vi "Read B.vi"(8 "Error In":errorcluster, 11 "NumericOperation in":refnum<class "NumericOperation.lvclass">) -> (0 "Error Out":errorcluster, 2 "B":dbl, 3 "NumericOperation out":refnum<class "NumericOperation.lvclass">)   [LabVIEW 2021, in "Calculator.lvlib" / "NumericOperation.lvclass"]
uses:
  NumericOperation.lvclass
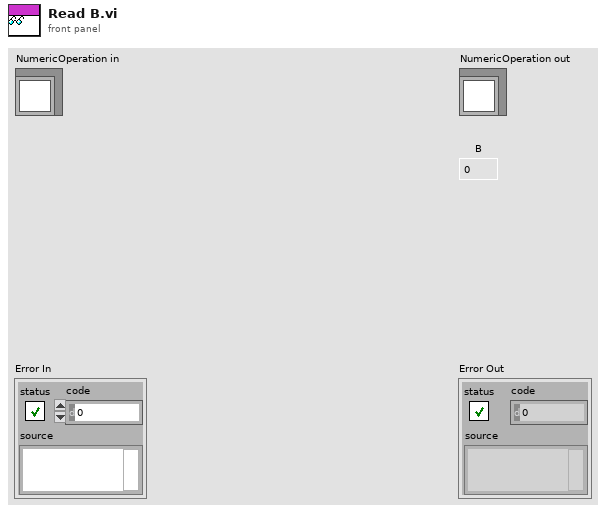
[diagram p1: front panel]
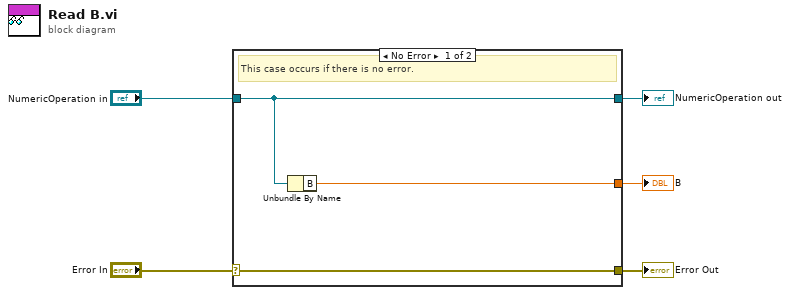
[diagram p0: block diagram]
diagram:
  n1 = case shown="No Error" "Error In" {
    selector: "Error In" -> [w8 w9]
    tunnel: [w8 w9] -> w4
    tunnel: [w7 w10] -> w2
    tunnel: "NumericOperation in" -> [w7 w10]
    tunnel: [w6 _] -> w1
    frame No Error {
      # "This case occurs if there is no error."
      n2 = Unbundle By Name(w7) -> ("B"=w6:dbl)
    }
    frame Error {
      # "This case occurs if there is any error"
    }
  }
  "Error Out" <- w4
  "NumericOperation out" <- w2
  "B" <- w1
